vi "backproject-worker.vi"(8 "Centre":i32[](array[numeric]), 9 "Write queue":refnum<queue>, 10 "Image Properties":T1, 11 "Work queue in":refnum<queue>) -> (1 "New Angle":dbl, 2 "finished angle":dbl, 3 "results":sgl[](array[numeric]))   [LabVIEW 2013]
uses:
  tags_cluster.ctl
  imagereconstruction/x64/Debug/labviewdll.dll
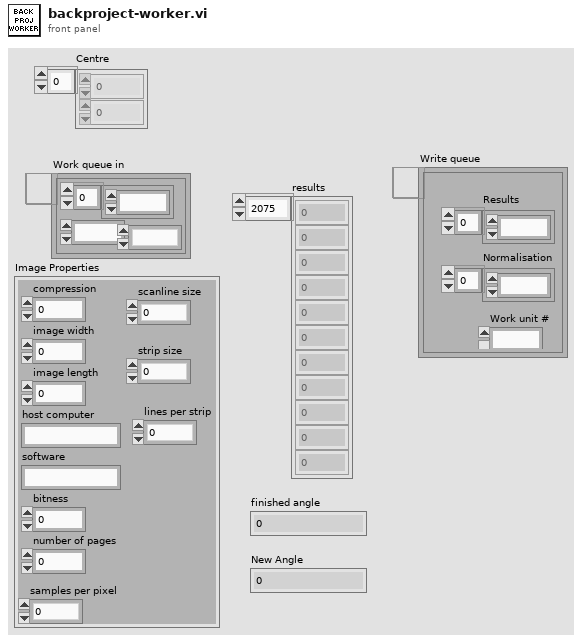
[diagram p1: front panel]
types:
  T1 = typedef "tags_cluster.ctl" = cluster{"compression":i32, "image width":i32, "image length":i32, "host computer":string, "software":string, "bitness":i32, "number of pages":i32, "samples per pixel":i32, "scanline size":i32, "strip size":i32, "lines per strip":i32}
  T2 = cluster{"results":sgl[], "normalisation":i32[], "Numeric":i32}
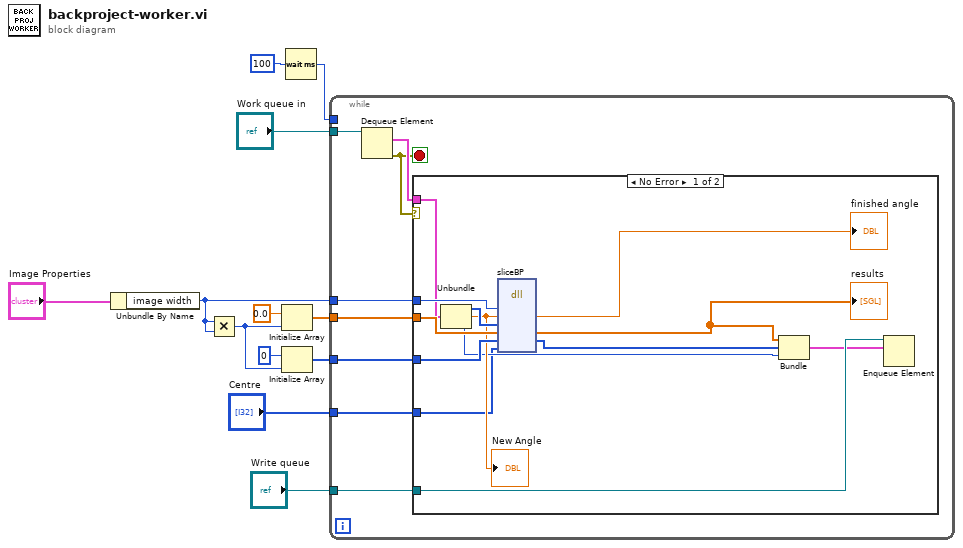
[diagram p0: block diagram]
diagram:
  n1 = Unbundle By Name("Image Properties") -> ("image width"=w12:i32)
  n2 = Multiply(x=w12, y=w12) -> (x*y=w11:i32)
  n3 = Initialize Array(sgl 0.0 ("element"), w11) -> (w8:sgl[])
  n4 = Initialize Array(0 ("element"), w11) -> (w6:i32[])
  n5 = Wait (ms)(milliseconds to wait=u32 100) -> (millisecond timer value=w10:u32)
  n6 = while {
    tunnel: "Work queue in" -> [w20]
    tunnel: w12 -> [w19]
    tunnel: w6 -> [w18]
    tunnel: w8 -> [w17]
    tunnel: w10 -> [_]
    tunnel: "Write queue" -> [w14]
    tunnel: "Centre" -> [w13]
    stop <- w15 stop-if-true
    n7 = Dequeue Element(queue=w20) -> (element=w16:cluster{u8[], dbl, "Numeric":i32}, error out=w15:errorcluster)  [unwired: 2 in, 2 out]
    n8 = case shown="No Error" w15 {
      tunnel: w19 -> [w33 _]
      tunnel: w18 -> [w32 _]
      tunnel: w17 -> [w31 _]
      tunnel: w16 -> [w30 _]
      tunnel: w14 -> [w27 _]
      tunnel: w13 -> [w21 _]
      frame No Error {
        n9 = Unbundle(w30) -> (w29:u8[], w28:dbl, "Numeric"=w22:i32)
        "New Angle" <- w28
        n10 = dll-call lib="D:/work/uni/FYP/reconrepo/imagereconstruction/x64/Debug/labviewdll.dll" fn="sliceBP"("w"=w33, "angle"=w28, "strip"=w29, "results"=w31, "normalisation"=w32, "centre"=w21) -> ("angle"=→"finished angle":dbl, "results"=w24:sgl[], "normalisation"=w23:i32[])  [unwired: 7 in, 2 out]
        "results" <- w24
        n11 = Bundle("results"=w24, "normalisation"=w23, "Numeric"=w22) -> (w25:T2)  [unwired: 1 in]
        n12 = Enqueue Element(queue=w27, element=w25) -> ()  [unwired: 2 in, 3 out]
      }
      frame Error {
      }
    }
  }
